vi "sendNavPosition.vi"(7 "vAccuracy":sgl, 8 "error in (no error)":errorcluster, 9 "hAccuracy":sgl, 10 "position":dbl[](array[numeric])=[0.0, 0.0, 0.0], 11 "pHandle":u32) -> (0 "error out":errorcluster, 3 "return type":i32)   [LabVIEW 2011, in "sbgLabView.lvlib"]
uses:
  sbgLabView.lvlib
  sbgMatLab.dll
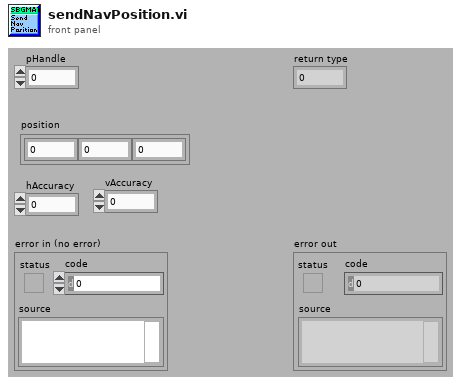
[diagram p1: front panel]
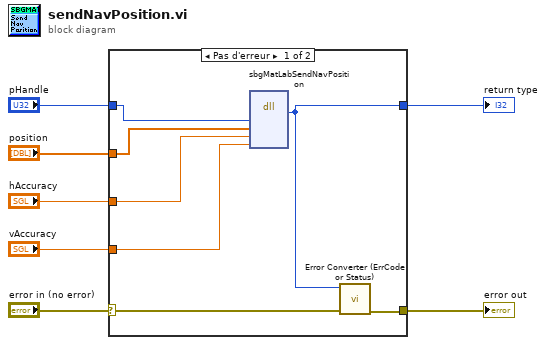
[diagram p0: block diagram]
diagram:
  n1 = case shown="Pas d'erreur" "error in (no error)" {
    selector: "error in (no error)" -> [w9 w15]
    tunnel: [w8 w15] -> w6
    tunnel: [w14 _] -> w5
    tunnel: "pHandle" -> [w13 _]
    tunnel: "position" -> [w12 _]
    tunnel: "hAccuracy" -> [w11 _]
    tunnel: "vAccuracy" -> [w10 _]
    frame No Error {
      n2 = dll-call lib="C:/SBG-Systems/remote/projects/software/projects/labviewExample/sbgLabView/sbgMatLab.*" fn="sbgMatLabSendNavPosition"("pHandle"=w13, "position"=w12, "hAccuracy"=w11, "vAccuracy"=w10) -> ("return type"=w14:i32)  [unwired: 7 in, 2 out]
      n3 = call "Error Converter (ErrCode or Status).vi"("error in (no error)"=w9, "error code"=w14) -> ("error out"=w8:errorcluster)  [unwired: 9 in]
    }
    frame Error {
    }
  }
  "return type" <- w5
  "error out" <- w6
